vi "SwerveCalculations.vi"(9 "J2X":dbl, 10 "J1Y":dbl, 11 "J1X":dbl) -> (0 "Magnitude 3":dbl, 1 "Magnitude 2":dbl, 2 "Magnitude 1":dbl, 3 "Magnitude 0":dbl, 4 "Wheel Angle 3":dbl, 5 "Wheel Angle 1":dbl, 6 "Wheel Angle 2":dbl, 7 "Wheel Angle 0":dbl)   [LabVIEW 2019]
panel:
  in  "Robot Width (in)":dbl=26.0
  in  "Robot Length (in)":dbl=26.0
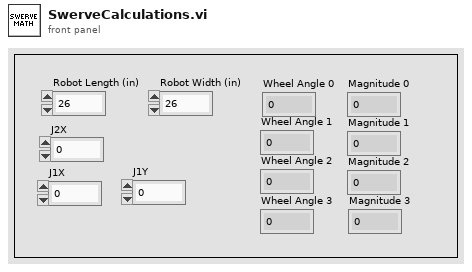
[diagram p1: front panel]
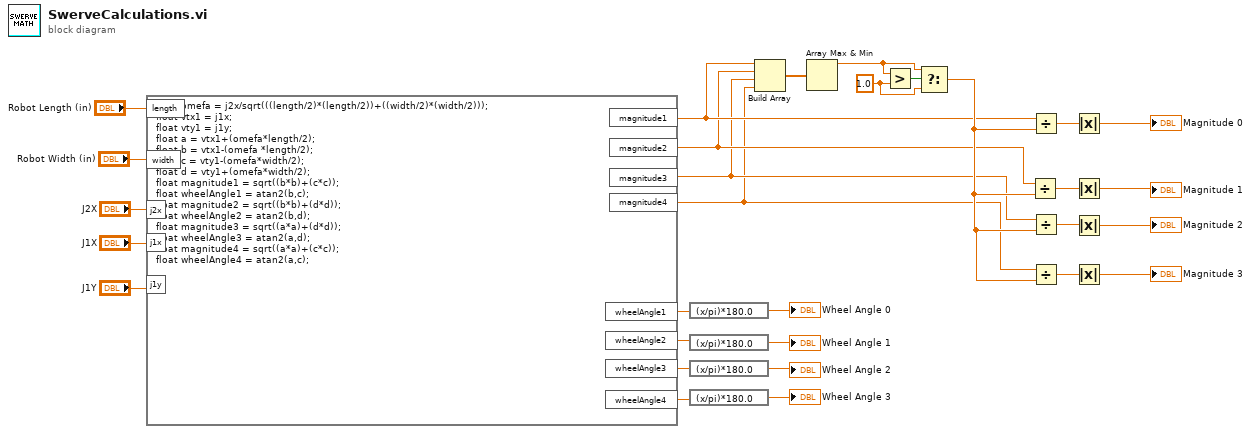
[diagram p0: block diagram]
diagram:
  w20 = 1.0 ("y")
  n1 = formula code="float omefa = j2x/sqrt(((length/2)*(length/2))+((width/2)*(width/2)));\nfloat vtx1 = j1x;\nfloat vty1 = j1y;\nfloat a = vtx1+(omefa*length/2);\nfloat b = vtx1-(omefa *length/2);\nfloat c = vty1-(omefa*width/2);\nfloat d = vty1+(omefa*width/2);\nfloat magnitude1 = sqrt((b*b)+(c*c));\nfloat wheelAngle1 = atan2(b,c);\nfloat magnitude2 = sqrt((b*b)+(d*d));\nfloat wheelAngle2 = atan2(b,d);\nfloat magnitude3 = sqrt((a*a)+(d*d));\nfloat wheelAngle3 = atan2(a,d);\nfloat magnitude4 = sqrt((a*a)+(c*c));\nfloat wheelAngle4 = atan2(a,c);"("length"="Robot Length (in)", "width"="Robot Width (in)", "j2x"="J2X", "j1y"="J1Y", "j1x"="J1X") -> ("wheelAngle1"=w6:dbl, "magnitude1"=w4:dbl, "magnitude2"=w3:dbl, "magnitude3"=w2:dbl, "magnitude4"=w1:dbl, "wheelAngle2"=w9:dbl, "wheelAngle3"=w11:dbl, "wheelAngle4"=w13:dbl)
  n2 = expression code="(x/pi)*180.0" ("radians to degrees")(w6) -> (→"Wheel Angle 0":dbl)
  n3 = expression code="(x/pi)*180.0" ("radians to degrees")(w9) -> (→"Wheel Angle 1":dbl)
  n4 = expression code="(x/pi)*180.0" ("radians to degrees")(w11) -> (→"Wheel Angle 2":dbl)
  n5 = expression code="(x/pi)*180.0" ("radians to degrees")(w13) -> (→"Wheel Angle 3":dbl)
  n6 = Build Array(w4, w3, w2, w1) -> (w5:dbl[])
  n7 = Array Max & Min(array=w5) -> (max value=w19:dbl)  [unwired: 3 out]
  n8 = Greater?(x=w19, y=w20) -> (0:w21:bool)
  n9 = Select(t=w19, s=w21, f=w20) -> (s? t:f=w15:dbl)
  n10 = Divide(x=w3, y=w15) -> (x/y=w17:dbl)
  n11 = Divide(x=w4, y=w15) -> (x/y=w18:dbl)
  n12 = Divide(x=w2, y=w15) -> (x/y=w16:dbl)
  n13 = Divide(x=w1, y=w15) -> (x/y=w14:dbl)
  n14 = Absolute Value(x=w18) -> (abs(x)=→"Magnitude 0":dbl)
  n15 = Absolute Value(x=w17) -> (abs(x)=→"Magnitude 1":dbl)
  n16 = Absolute Value(x=w16) -> (abs(x)=→"Magnitude 2":dbl)
  n17 = Absolute Value(x=w14) -> (abs(x)=→"Magnitude 3":dbl)
